vi "Parse Test Configs.vi"(0 "TestConfigurations Element":refnum<k20>, 11 "error in":errorcluster) -> (6 "Test Configurations":T3(array[cluster]) {"Test Ranking" items=["Low", "Normal", "High"]}, 15 "error out":errorcluster)   [LabVIEW 2020]
uses:
  <vilib>/addons/analyzer/_analyzerctrls.llb/VIAnCtl TestRanking.ctl
  <vilib>/addons/analyzer/_analyzerctrls.llb/VIAnCtl Config Control Value.ctl
  <vilib>/xml/Close Reference(Node).vi
  <vilib>/xml/NI_XML.lvlib
  <resource>/objmgr/DOMUserDefRef.rc
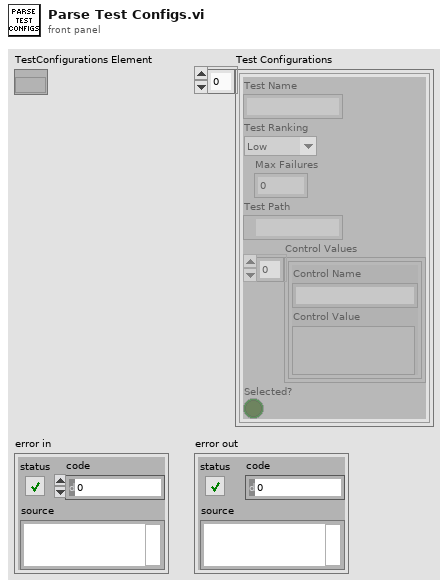
[diagram p1: front panel]
types:
  T1 = typedef "VIAnCtl TestRanking.ctl" = u16
  T2 = typedef "VIAnCtl Config Control Value.ctl" = cluster{"Control Name":string, "Control Value":variant}
  T3 = cluster{"Test Name":string, "Test Ranking":T1, "Max Failures":u32, "Test Path":path, "Control Values":T2[], "Selected?":bool}[]
  T4 = cluster{"Test Name":string, "Test Ranking":T1, "Max Failures":u32, "Test Path":path, "Control Values":T2[], "Selected?":bool}
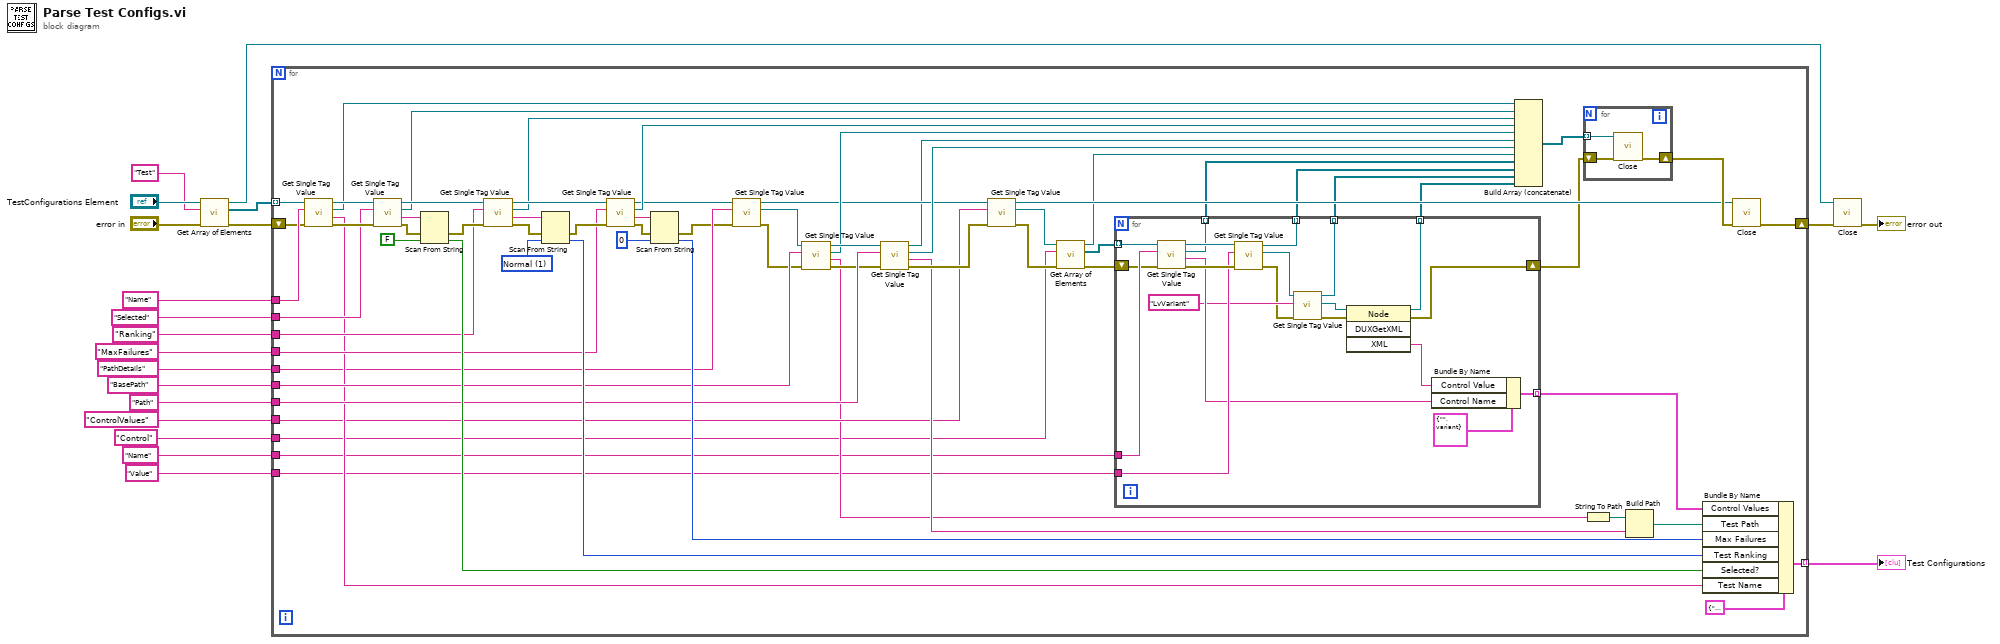
[diagram p0: block diagram]
diagram:
  n1 = call <vilib>:"Get Array of Elements.vi"("error in (no error)"="error in", "Tag Name"="Test", "Refnum in"="TestConfigurations Element") -> ("error out"=w9:errorcluster, "Array Of Elements"=w8:refnum<k20>[], "Refnum out"=w7:refnum<k20>)  [unwired: 6 in]
  n2 = for {
    tunnel: w8 -> [w88] mode=indexing
    tunnel: "Name" ("Tag Name") -> [w87]
    shift-right: [w60] -> w11
    shift-left: w9 -> [w86]
    tunnel: "Selected" ("Tag Name") -> [w82]
    tunnel: "Ranking" ("Tag Name") -> [w76]
    tunnel: "MaxFailures" ("Tag Name") -> [w70]
    tunnel: "PathDetails" ("Tag Name") -> [w44]
    tunnel: "BasePath" ("Tag Name") -> [w66]
    tunnel: "Path" ("Tag Name") -> [w64]
    tunnel: "ControlValues" ("Tag Name") -> [w38]
    tunnel: [w61] -> w12 mode=indexing
    tunnel: "Name" ("Tag Name") -> [w34]
    tunnel: "Value" ("Tag Name") -> [w33]
    tunnel: "Control" ("Tag Name") -> [w22]
    w73 = T1 1 items=["Low", "Normal", "High"] ("Test Ranking")
    n3 = call <vilib>:"Get Single Tag Value.vi"("Error In"=w86, "Tag Name"=w87, "Element In"=w88) -> ("Error Out"=w83:errorcluster, "Tag Value"=w59:string, "Tag Reference"=w55:refnum<k20>, "Element Out"=w84:refnum<k20>)  [unwired: 5 in]
    n4 = call <vilib>:"Get Single Tag Value.vi"("Error In"=w83, "Tag Name"=w82, "Element In"=w84) -> ("Error Out"=w80:errorcluster, "Tag Value"=w58:string, "Tag Reference"=w54:refnum<k20>, "Element Out"=w81:refnum<k20>)  [unwired: 5 in]
    n5 = Scan From String(input string=w58, error in=w80, default 1=FALSE) -> (error out=w79:errorcluster, output 1=w77:bool)  [unwired: 2 in, 2 out]
    n6 = call <vilib>:"Get Single Tag Value.vi"("Error In"=w79, "Tag Name"=w76, "Element In"=w81) -> ("Error Out"=w75:errorcluster, "Tag Value"=w56:string, "Tag Reference"=w53:refnum<k20>, "Element Out"=w71:refnum<k20>)  [unwired: 5 in]
    n7 = Scan From String(input string=w56, error in=w75, default 1=w73) -> (error out=w72:errorcluster, output 1=w74:T1)  [unwired: 2 in, 2 out]
    n8 = call <vilib>:"Get Single Tag Value.vi"("Error In"=w72, "Tag Name"=w70, "Element In"=w71) -> ("Error Out"=w69:errorcluster, "Tag Value"=w57:string, "Tag Reference"=w52:refnum<k20>, "Element Out"=w47:refnum<k20>)  [unwired: 5 in]
    n9 = Scan From String(input string=w57, error in=w69, default 1=u32 0 ("Max Failures")) -> (error out=w43:errorcluster, output 1=w67:u32)  [unwired: 2 in, 2 out]
    n10 = call <vilib>:"Get Single Tag Value.vi"("Error In"=w43, "Tag Name"=w44, "Element In"=w47) -> ("Error Out"=w46:errorcluster, "Tag Reference"=w45:refnum<k20>, "Element Out"=w40:refnum<k20>)  [unwired: 5 in, 1 out]
    n11 = call <vilib>:"Get Single Tag Value.vi"("Error In"=w46, "Tag Name"=w66, "Element In"=w45) -> ("Error Out"=w63:errorcluster, "Tag Value"=w36:string, "Tag Reference"=w51:refnum<k20>, "Element Out"=w65:refnum<k20>)  [unwired: 5 in]
    n12 = call <vilib>:"Get Single Tag Value.vi"("Error In"=w63, "Tag Name"=w64, "Element In"=w65) -> ("Error Out"=w62:errorcluster, "Tag Value"=w42:string, "Tag Reference"=w50:refnum<k20>, "Element Out"=w37:refnum<k20>)  [unwired: 5 in]
    n13 = call <vilib>:"Get Single Tag Value.vi"("Error In"=w62, "Tag Name"=w38, "Element In"=w40) -> ("Error Out"=w26:errorcluster, "Tag Reference"=w27:refnum<k20>, "Element Out"=w39:refnum<k20>)  [unwired: 5 in, 1 out]
    n14 = call <vilib>:"Get Array of Elements.vi"("error in (no error)"=w26, "Tag Name"=w22, "Refnum in"=w27) -> ("error out"=w24:errorcluster, "Array Of Elements"=w25:refnum<k20>[], "Refnum out"=w23:refnum<k20>)  [unwired: 6 in]
    n15 = for {
      tunnel: w34 -> [w108]
      tunnel: w33 -> [w105]
      tunnel: [w104] -> w32 mode=indexing
      tunnel: [w103] -> w31 mode=indexing
      tunnel: [w90] -> w30 mode=indexing
      tunnel: [w100] -> w29 mode=indexing
      tunnel: w25 -> [w99] mode=indexing
      shift-right: [w91] -> w28
      shift-left: w24 -> [w98]
      tunnel: [w89] -> w21 mode=indexing
      n16 = call <vilib>:"Get Single Tag Value.vi"("Error In"=w98, "Tag Name"=w108, "Element In"=w99) -> ("Error Out"=w106:errorcluster, "Tag Value"=w102:string, "Tag Reference"=w104:refnum<k20>, "Element Out"=w107:refnum<k20>)  [unwired: 5 in]
      n17 = call <vilib>:"Get Single Tag Value.vi"("Error In"=w106, "Tag Name"=w105, "Element In"=w107) -> ("Error Out"=w94:errorcluster, "Tag Reference"=w97:refnum<k20>, "Element Out"=w103:refnum<k20>)  [unwired: 5 in, 1 out]
      n18 = call <vilib>:"Get Single Tag Value.vi"("Error In"=w94, "Tag Name"="LvVariant", "Element In"=w97) -> ("Error Out"=w95:errorcluster, "Tag Reference"=w93:refnum<k20>, "Element Out"=w90:refnum<k20>)  [unwired: 5 in, 1 out]
      n19 = invoke class="Node" method="DUXGetXML"(reference=w93, error in=w95) -> (reference out=w89:refnum<k20>, error out=w91:errorcluster, "XML"=w92:string)  [unwired: 2 in, 1 out]
      n20 = Bundle By Name(cluster=T2 {"Control Name"="", "Control Value"=variant(string "")} ("Config Control Value"), "Control Value"=w92, "Control Name"=w102) -> (w100:T2)
    }
    n21 = Build Array (concatenate)(w55, w54, w53, w52, w51, w37, w50, w23, w32, w31, w30, w21) -> (w49:refnum<k20>[])
    n22 = for {
      tunnel: w49 -> [w111] mode=indexing
      shift-right: [w110] -> w48
      shift-left: w28 -> [w109]
      n23 = call-poly <vilib>:"Close.vi"("error in (no error)"=w109, "node"=w111) -> ("error out"=w110:errorcluster)  [unwired: 7 in]
    }
    n24 = String To Path(string=w36) -> (path=w35:path)
    n25 = Build Path(base path=w35, name or relative path=w42) -> (appended path=w41:path)
    n26 = Bundle By Name(cluster=T4 {"Test Name"="", "Test Ranking"=0, "Max Failures"=0, "Test Path"=path "", "Control Values"=[], "Selected?"=FALSE} ("Cluster"), "Control Values"=w29, "Test Path"=w41, "Max Failures"=w67, "Test Ranking"=w74, "Selected?"=w77, "Test Name"=w59) -> (w61:T4)
    n27 = call-poly <vilib>:"Close.vi"("error in (no error)"=w48, "node"=w39) -> ("error out"=w60:errorcluster)  [unwired: 7 in]
  }
  "Test Configurations" <- w12
  n28 = call-poly <vilib>:"Close.vi"("error in (no error)"=w11, "node"=w7) -> ("error out"=→"error out":errorcluster)  [unwired: 7 in]
